vi "FTW-STR-Display-Bytes.vi"(0 "Bytes":i64 format="%d bytes", 1 "Display Format":T1) -> (2 "Display":string)   [LabVIEW 2012]
uses:
  FTW-STR-DisplayFormat-Bytes.ctl
panel:
  # "Inputs"
  # "Outputs"
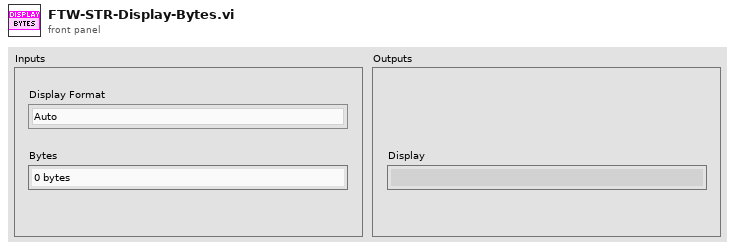
[diagram p1: front panel]
types:
  T1 = typedef "FTW-STR-DisplayFormat-Bytes.ctl" = enum16{"Auto", "Plain Bytes", "000 bytes", "0.00kB", "0.00MB", "0.00GB", "0.00TB", "Transfer Rate"}
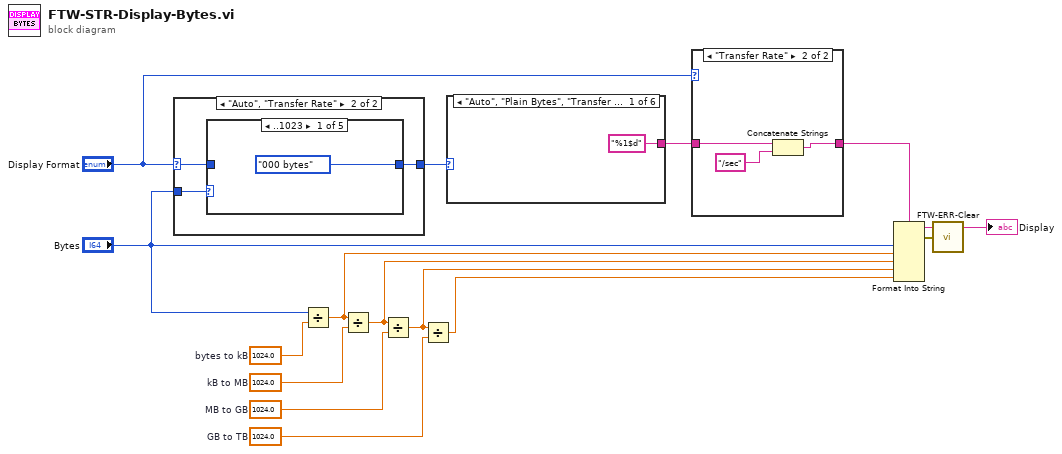
[diagram p0: block diagram]
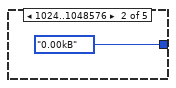
[diagram p4: hidden frame]
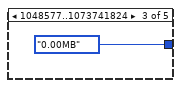
[diagram p5: hidden frame]
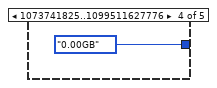
[diagram p6: hidden frame]
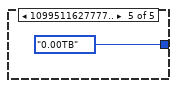
[diagram p7: hidden frame]
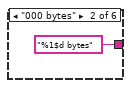
[diagram p8: hidden frame]
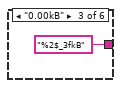
[diagram p9: hidden frame]
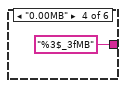
[diagram p10: hidden frame]
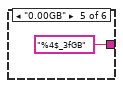
[diagram p11: hidden frame]
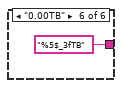
[diagram p12: hidden frame]
diagram:
  w11 = 1024.0  # GB to TB
  w12 = 1024.0  # MB to GB
  w13 = 1024.0  # kB to MB
  w14 = 1024.0  # bytes to kB
  n1 = case shown="\"Auto\", \"Transfer Rate\"" "Display Format" {
    selector: "Display Format" -> [w16 w18]
    tunnel: "Bytes" -> [_ w19]
    tunnel: [w16 w17] -> w4
    frame Default {
    }
    frame "Auto", "Transfer Rate" {
      n2 = case shown="..1023" w19 {
        tunnel: w18 -> [_ _ _ _ _]
        tunnel: [FTW-STR-DisplayFormat-Bytes."000 bytes" ("Display Style") FTW-STR-DisplayFormat-Bytes."0.00kB" ("Display Style") FTW-STR-DisplayFormat-Bytes."0.00MB" ("Display Style") FTW-STR-DisplayFormat-Bytes."0.00GB" ("Display Style") FTW-STR-DisplayFormat-Bytes."0.00TB" ("Display Style")] -> w17
        frame ..1023 {
        }
        frame 1024..1048576 {
        }
        frame 1048577..1073741824 {
        }
        frame 1073741825..1099511627776 {
        }
        frame 1099511627777.. {
        }
      }
    }
  }
  n3 = Divide(x="Bytes", y=w14) -> (x/y=w10:dbl)
  n4 = Divide(x=w10, y=w13) -> (x/y=w9:dbl)
  n5 = Divide(x=w9, y=w12) -> (x/y=w8:dbl)
  n6 = Divide(x=w8, y=w11) -> (x/y=w7:dbl)
  n7 = case shown="\"Auto\", \"Plain Bytes\", \"Transfer Rate\"" w4 {
    tunnel: ["%1$d" "%1$d bytes" "%2$_3fkB" "%3$_3fMB" "%4$_3fGB" "%5$_3fTB"] -> w1
    frame "Auto", "Plain Bytes", "Transfer Rate" {
    }
    frame "000 bytes" {
    }
    frame "0.00kB" {
    }
    frame "0.00MB" {
    }
    frame "0.00GB" {
    }
    frame "0.00TB" {
    }
  }
  n8 = case shown="\"Transfer Rate\"" "Display Format" {
    tunnel: [w31 w32] -> w2
    tunnel: w1 -> [w31 w34]
    frame Default {
    }
    frame "Transfer Rate" {
      n9 = Concatenate Strings(w34, "/sec" ("string")) -> (w32:string)
    }
  }
  n10 = Format Into String(format string=w2, "Bytes", w10, w9, w8, w7) -> (resulting string=→"Display":string, error out=w15:errorcluster)  [unwired: 2 in]
  n11 = call "FTW-ERR-Clear.vi"("error to snuff"=w15) -> ()  [unwired: 1 out]
